vi "Calibration Due date - UI.vi"(0 "Calibration Info":T1={"Parameter"="DMM", "Last_ST_Date"="12/27/2011", "ST_Due_Date"="12/28/2011", "Corrections"="1"}, 7 "Calibrate All":bool) -> (4 "Due Date":string, 6 "Calibrated Date":string, 8 "Modified":bool)   [LabVIEW 2010]
uses:
  Calibration dates.ctl
panel:
  out "Welcome String":string
  in  "Exit":bool
  in  "Next Calibration Date":timestamp=timestamp(3296822614.6226506 s since 1904-01-01) format="%<%x>T"
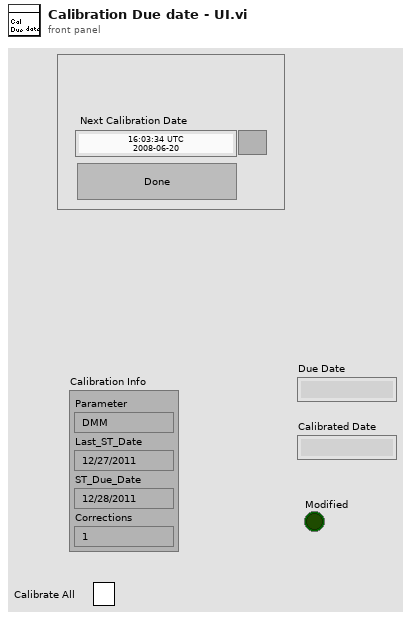
[diagram p1: front panel]
types:
  T1 = typedef "Calibration dates.ctl" = cluster{"Parameter":string, "Last_ST_Date":string, "ST_Due_Date":string, "Corrections":string}
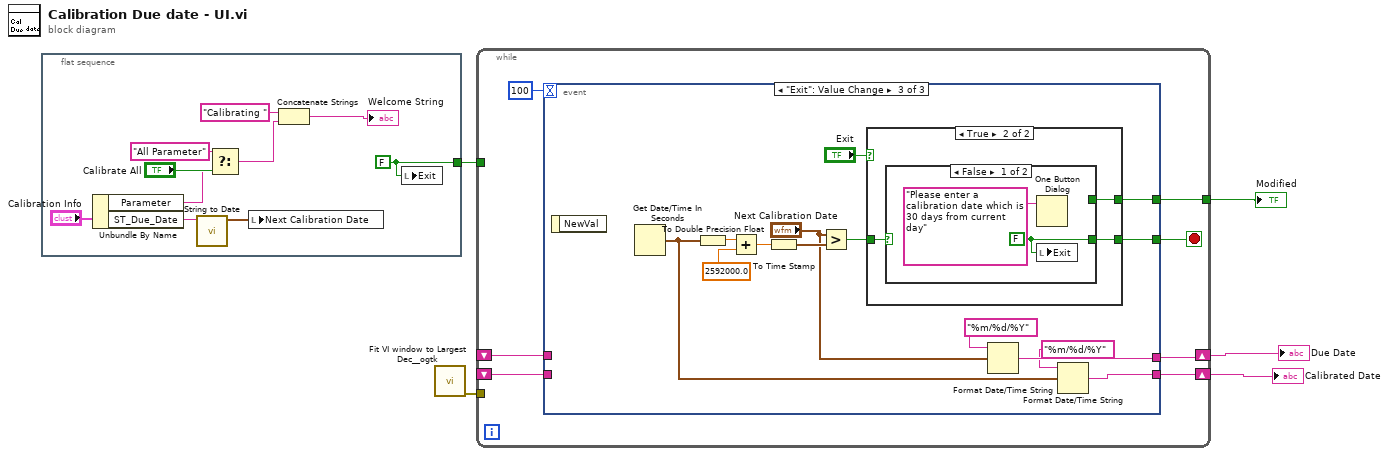
[diagram p0: block diagram]
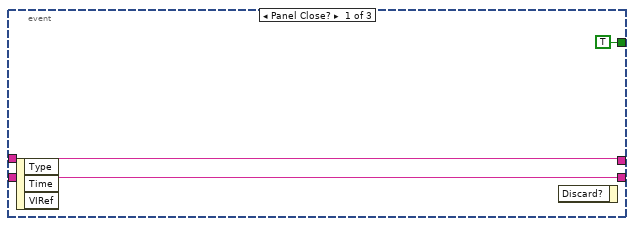
[diagram p2: hidden frame]
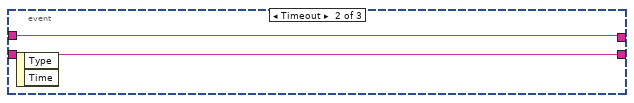
[diagram p3: hidden frame]
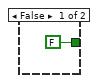
[diagram p4: hidden frame]
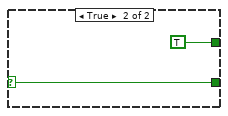
[diagram p5: hidden frame]
diagram:
  n1 = flat-sequence {
    tunnel: [w15] -> w4
    frame #0 {
      w15 = FALSE ("Exit")
      n2 = Unbundle By Name("Calibration Info") -> ("Parameter"=w9:string, "ST_Due_Date"=w13:string)
      n3 = call "String to Date.vi"("Cal Due Date"=w13) -> ("time stamp"=w12:timestamp)  [unwired: 10 in]
      n4 = Select(t="All Parameter", s="Calibrate All", f=w9) -> (s? t:f=w7:string)
      n5 = local write "Next Calibration Date"(w12) -> ()
      n6 = Concatenate Strings("Calibrating " ("string"), w7) -> (→"Welcome String":string)
      n7 = local write "Exit"(w15) -> ()
    }
  }
  n8 = call <userlib>:"Fit VI window to Largest Dec__ogtk.vi"() -> ("error out"=w5:errorcluster)  [unwired: 6 in, 1 out]
  n9 = while {
    tunnel: w5 -> [_]
    tunnel: w4 -> [_]
    shift-right: [w21] -> w2
    shift-left: _ -> [w19]
    shift-right: [w20] -> w3
    shift-left: _ -> [w18]
    tunnel: [w16] -> w1
    stop <- w22 stop-if-true
    n10 = event shown="[2] \"Exit\": Value Change" {
      selector: _ -> [_ _ _]
      dyn-events: _ -> [_ _ _]
      timeout: 100 -> [_ _ _]
      tunnel: [w25 w27 w32] -> w21
      tunnel: [w24 w26 w28] -> w20
      tunnel: w19 -> [w25 w27 _]
      tunnel: w18 -> [w24 w26 _]
      tunnel: [TRUE _ w40] -> w22
      tunnel: [_ _ w31] -> w16
      event Panel Close? {
        n11 = event-data() -> ()  [unwired: 1 in, 3 out]
        n12 = event-data() -> ()  [unwired: 2 in, 1 out]
      }
      event Timeout {
        n13 = event-data() -> ()  [unwired: 1 in, 2 out]
      }
      event "Exit": Value Change {
        n14 = event-data() -> ()  [unwired: 1 in, 1 out]
        n15 = Get Date/Time In Seconds() -> (seconds since 1Jan1904=w29:timestamp)
        n16 = To Double Precision Float(number=w29) -> (double precision float=w38:dbl)
        n17 = Add(x=w38, y=2592000.0) -> (x+y=w36:dbl)
        n18 = To Time Stamp(1:w36) -> (0:w35:timestamp)
        n19 = Greater?(x="Next Calibration Date", y=w35) -> (0:w41:bool)
        n20 = case shown="True" "Exit" {
          tunnel: [FALSE ("Exit") w44] -> w40
          tunnel: w41 -> [_ w45]
          tunnel: [_ w43] -> w31
          frame False {
          }
          frame True {
            n21 = case shown="False" w45 {
              selector: w45 -> [_ w49]
              tunnel: [w47 w49] -> w44
              tunnel: [_ TRUE ("Exit")] -> w43
              frame False {
                w47 = FALSE
                n22 = One Button Dialog(message="Please enter a calibration date which is 30 days from current day") -> ()  [unwired: 1 in, 1 out]
                n23 = local write "Exit"(w47) -> ()
              }
              frame True {
              }
            }
          }
        }
        n24 = Format Date/Time String(time format string (%c)="%m/%d/%Y", seconds (now)="Next Calibration Date") -> (date/time string=w32:string)  [unwired: 1 in]
        n25 = Format Date/Time String(time format string (%c)="%m/%d/%Y", seconds (now)=w29) -> (date/time string=w28:string)  [unwired: 1 in]
      }
    }
  }
  "Due Date" <- w2
  "Calibrated Date" <- w3
  "Modified" <- w1
